vi "test6-AsyncMessageWithReplyWithError.vi"(8 "error in (no error)":errorcluster, 11 "TestCase in":refnum<class "testcase-CSMMessage.lvclass">) -> (0 "error out":errorcluster, 3 "TestCase out":refnum<class "testcase-CSMMessage.lvclass">)   [LabVIEW 2017, in "testcase-CSMMessage.lvclass"]
uses:
  testcase-CSMMessage.lvclass
  948582eb-d69d-4bf1-bb36-25d021f5d5c5.vi
  src/user.lib/_NEVSTOP/Communicable State Machine(CSM)/AdvanceAPI/CSM - Make String Arguments Safe.vi
  src/user.lib/_NEVSTOP/Communicable State Machine(CSM)/AdvanceAPI/CSM - Keywords.vi
  <vilib>/addons/_JKI Toolkits/VI Tester/TestCase.llb/TestCase.lvclass
  src/user.lib/_NEVSTOP/Communicable State Machine(CSM)/Communicable State Machine.lvlib
  C:/Program Files (x86)/National Instruments/LabVIEW 2017/vi.lib/addons/_JKI Toolkits/VI Tester/TestCase.llb/TestCase.lvclass
panel:
  out "Loop Count":i32
  out "debug message":string
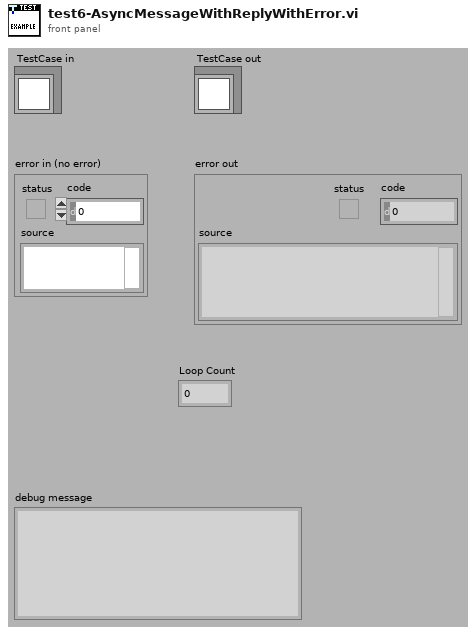
[diagram p1: front panel]
types:
  T1 = cluster{"Arguments":string, "Response":string, "error":errorcluster}
  T2 = cluster{"status":bool, "code":bool, "source":bool}
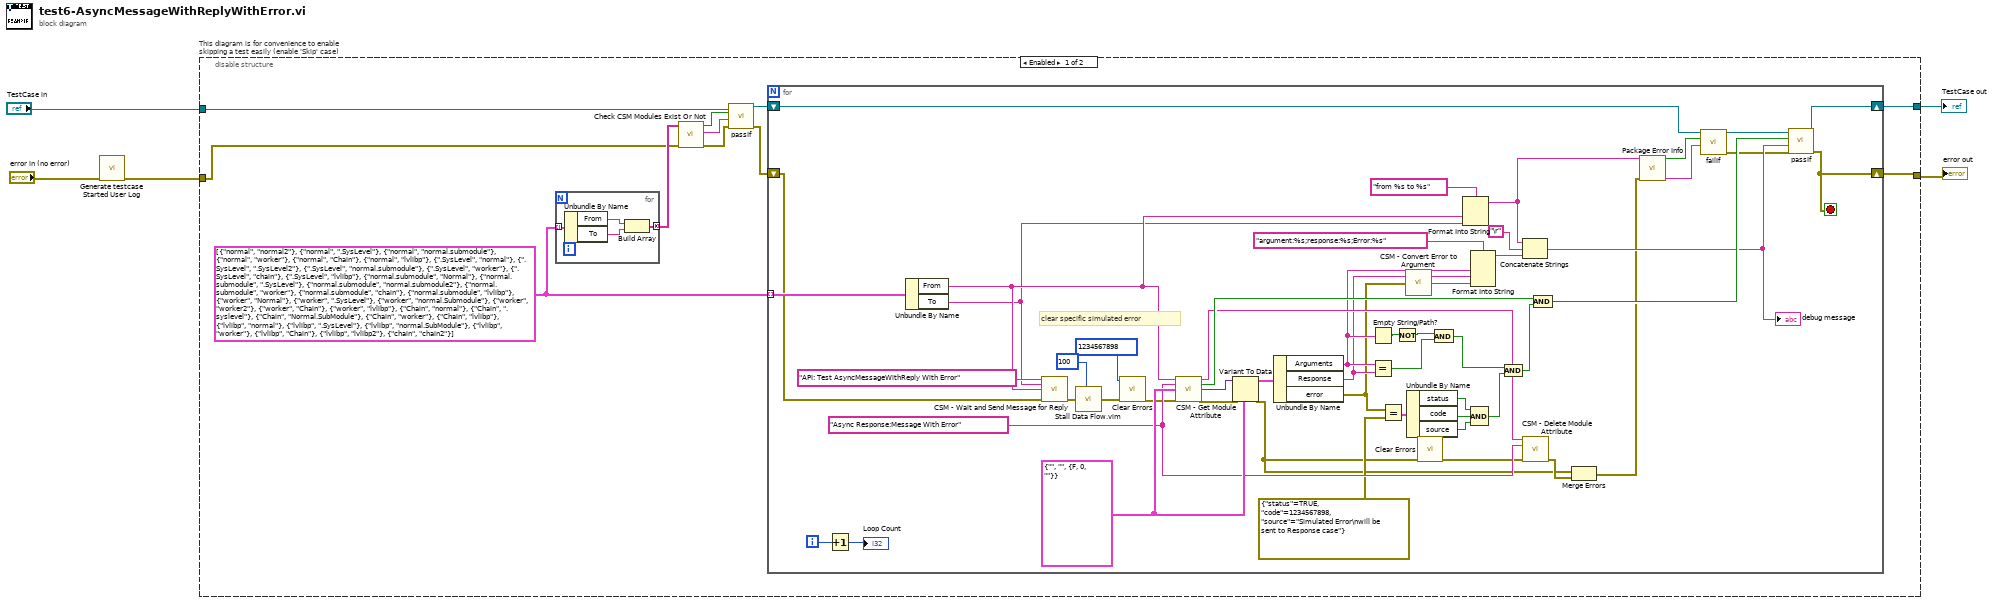
[diagram p0: block diagram]
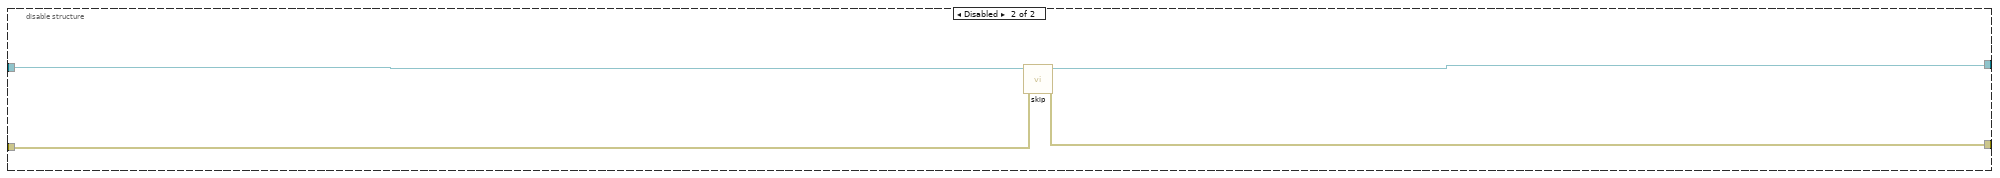
[diagram p2: hidden frame]
diagram:
  n1 = call "Generate testcase Started User Log.vi"("Error In"="error in (no error)") -> ("error out"=w1:errorcluster)  [unwired: 10 in]
  n2 = disable-structure "This diagram is for convenience to enable skipping a test easily (enable 'Skip' case)" shown="Enabled" {
    disable-tunnel: "TestCase in" -> [w11 w76]
    disable-tunnel: [w7 w74] -> w2
    disable-tunnel: [w6 w75] -> w4
    disable-tunnel: w1 -> [w9 w73]
    frame Enabled {
      w12 = cluster{"From":string, "To":string}[] [{"From"="normal", "To"="normal2"}, {"From"="normal", "To"=".SysLevel"}, {"From"="normal", "To"="normal.submodule"}, {"From"="normal", "To"="worker"}, {"From"="normal", "To"="Chain"}, {"From"="normal", "To"="lvlibp"}, {"From"=".SysLevel", "To"="normal"}, {"From"=".SysLevel", "To"=".SysLevel2"}, {"From"=".SysLevel", "To"="normal.submodule"}, {"From"=".SysLevel", "To"="worker"}, {"From"=".SysLevel", "To"="chain"}, {"From"=".SysLevel", "To"="lvlibp"}, {"From"="normal.submodule", "To"="Normal"}, {"From"="normal.submodule", "To"=".SysLevel"}, {"From"="normal.submodule", "To"="normal.submodule2"}, {"From"="normal.submodule", "To"="worker"}, {"From"="normal.submodule", "To"="chain"}, {"From"="normal.submodule", "To"="lvlibp"}, {"From"="worker", "To"="Normal"}, {"From"="worker", "To"=".SysLevel"}, {"From"="worker", "To"="normal.Submodule"}, {"From"="worker", "To"="worker2"}, {"From"="worker", "To"="Chain"}, {"From"="worker", "To"="lvlibp"}, {"From"="Chain", "To"="normal"}, {"From"="Chain", "To"=".syslevel"}, {"From"="Chain", "To"="Normal.SubModule"}, {"From"="Chain", "To"="worker"}, {"From"="Chain", "To"="lvlibp"}, {"From"="lvlibp", "To"="normal"}, {"From"="lvlibp", "To"=".SysLevel"}, {"From"="lvlibp", "To"="normal.SubModule"}, {"From"="lvlibp", "To"="worker"}, {"From"="lvlibp", "To"="Chain"}, {"From"="lvlibp", "To"="lvlibp2"}, {"From"="chain", "To"="chain2"}]
      n3 = for {
        tunnel: w12 -> [w20] mode=indexing
        tunnel: [w17] -> w15 mode=concatenating
        n4 = Unbundle By Name(w20) -> ("From"=w19:string, "To"=w18:string)
        n5 = Build Array(w19, w18) -> (w17:string[])
      }
      n6 = call "Check CSM Modules Exist Or Not.vi"("error in"=w9, "CSM names in"=w15) -> ("error out"=w13:errorcluster, "Debug string"=w14:string, "All Modules Exist?"=w16:bool)  [unwired: 7 in]
      n7 = call-dynamic "passIf.vi"("error in (no error)"=w13, "message (\"\")"=w14, "pass"=w16, "TestCase in"=w11) -> ("error out"=w8:errorcluster, "TestCase out"=w10:refnum<class "testcase-CSMMessage.lvclass">)  [unwired: 6 in]
      n8 = for {
        tunnel: w12 -> [w63] mode=indexing
        shift-right: [w72] -> w7
        shift-left: w10 -> [w25]
        shift-right: [w48] -> w6
        shift-left: w8 -> [w32]
        i -> [w36]
        stop <- w48 stop-if-true
        w69 = T1 {"Arguments"="", "Response"="", "error"={"status"=FALSE, "code"=0, "source"=""}}
        w60 = "Async Response:Message With Error" ("State")
        # "clear specific simulated error"
        n9 = Increment(x=w36) -> (x+1=→"Loop Count":i32)
        n10 = Unbundle By Name(w63) -> ("From"=w40:string, "To"=w39:string)
        n11 = call "CSM - Wait and Send Message for Reply.vi"("State"="API: Test AsyncMessageWithReply With Error", "Arguments (\"\")"=w39, "Target Module"=w40, "Error In (No Error)"=w32) -> ("error out"=w33:errorcluster)  [unwired: 8 in, 3 out]
        n12 = call "Stall Data Flow.vim"("value in"=w33, "milliseconds to wait"=u32 100) -> ("value out"=w37:errorcluster)  [unwired: 1 out]
        n13 = call <vilib>:"Clear Errors.vi"("error in (no error)"=w37, "specific error code to clear (0: all)"=1234567898) -> ("error out"=w38:errorcluster)  [unwired: 4 in, 1 out]
        n14 = call "CSM - Get Module Attribute.vi"("CSM Name"=w40, "Attribute"=w60, "Default Value (Empty Variant)"=w69, "Error In"=w38) -> ("CSM Name (Dup)"=w61:string, "Found"=w66:bool, "Value"=w68:variant, "error out"=w70:errorcluster)  [unwired: 7 in, 1 out]
        n15 = Variant To Data(error in=w70, type=w69, Variant=w68) -> (data=w67:T1, error out=w29:errorcluster)
        n16 = Unbundle By Name(w67) -> ("Arguments"=w55:string, "Response"=w54:string, "error"=w47:errorcluster)
        n17 = Empty String/Path?(string/path=w55) -> (empty?=w59:bool)
        n18 = Equal?(x=w55, y=w54) -> (x = y?=w57:bool)
        n19 = Equal?(x=w47, y=errorcluster {"status"=TRUE, "code"=1234567898, "source"="Simulated Error\nwill be sent to Response case"} ("error out")) -> (x = y?=w45:T2)
        n20 = Not(x=w59) -> (.not. x?=w58:bool)
        n21 = call "CSM - Convert Error to Argument.vi"("Error"=w47) -> ("Argument"=w53:string)  [unwired: 4 in]
        n22 = Unbundle By Name(w45) -> ("status"=w44:bool, "code"=w43:bool, "source"=w42:bool)
        n23 = call <vilib>:"Clear Errors.vi"("error in (no error)"=w29) -> ("error out"=w49:errorcluster)  [unwired: 5 in, 1 out]
        n24 = And(x=w58, y=w57) -> (x .and. y?=w56:bool)
        n25 = Format Into String(format string="from %s to %s", w40, w39) -> (resulting string=w21:string)  [unwired: 2 in, 1 out]
        n26 = Format Into String(format string="argument:%s;response:%s;Error:%s", w55, w54, w53) -> (resulting string=w52:string)  [unwired: 2 in, 1 out]
        n27 = Compound Arithmetic op=AND(w44, w43, w42) -> (w41:bool)
        n28 = And(x=w56, y=w41) -> (x .and. y?=w65:bool)
        n29 = Concatenate Strings(w21, "\r", w52) -> (w28:string)
        "debug message" <- w28
        n30 = call "CSM - Delete Module Attribute.vi"("CSM Name"=w61, "Attribute"=w60, "Error In"=w49) -> ("error out"=w30:errorcluster)  [unwired: 9 in, 3 out]
        n31 = And(x=w66, y=w65) -> (x .and. y?=w64:bool)
        n32 = Merge Errors(w29, w30) -> (w22:errorcluster)
        n33 = call "Package Error Info.vi"("error in"=w22, "String in"=w21) -> ("packed error info out"=w26:string, "error status"=w27:bool)  [unwired: 8 in]
        n34 = call-dynamic "failIf.vi"("message (\"\")"=w26, "fail"=w27, "TestCase in"=w25) -> ("error out"=w23:errorcluster, "TestCase out"=w24:refnum<class "testcase-CSMMessage.lvclass">)  [unwired: 7 in]
        n35 = call-dynamic "passIf.vi"("error in (no error)"=w23, "message (\"\")"=w28, "pass"=w64, "TestCase in"=w24) -> ("error out"=w48:errorcluster, "TestCase out"=w72:refnum<class "testcase-CSMMessage.lvclass">)  [unwired: 6 in]
      }
    }
    frame Disabled {
      # "skip test result while test is under development"
      n36 = call <vilib>:"skip.vi"("error in (no error)"=w73, "TestCase in"=w76) -> ("error out"=w75:errorcluster, "TestCase out"=w74:refnum<class "testcase-CSMMessage.lvclass">)  [unwired: 8 in]
    }
  }
  "error out" <- w4
  "TestCase out" <- w2
